vi "picoquant_write_processing_tasks.vi"(8 "error in (no error)":errorcluster, 10 "processing tasks":T1, 11 "picoquant_generic in":refnum<class "picoquant_generic.lvclass">) -> (0 "error out":errorcluster, 3 "picoquant_generic out":refnum<class "picoquant_generic.lvclass">)   [LabVIEW 2015, in "picoquant_generic.lvclass"]
uses:
  picoquant_generic.lvclass
  processing_tasks_tdef.ctl
  picoquant_generic.lvclass/picoquant_generic.ctl
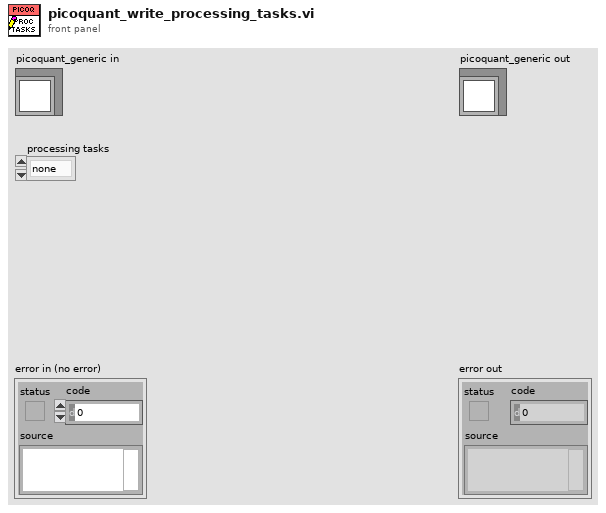
[diagram p1: front panel]
types:
  T1 = typedef "processing_tasks_tdef.ctl" = enum16{"none", "correlate", "histogram"}
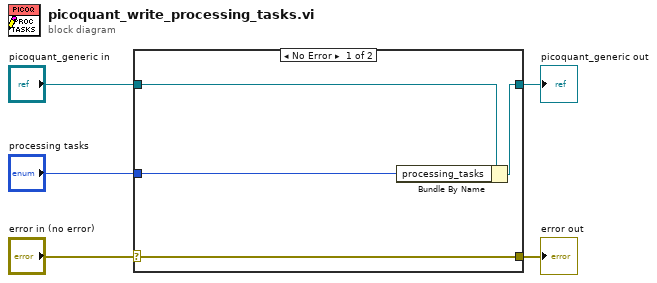
[diagram p0: block diagram]
diagram:
  n1 = case shown="No Error" "error in (no error)" {
    selector: "error in (no error)" -> [w9 w10]
    tunnel: [w9 w10] -> w4
    tunnel: [w7 w11] -> w2
    tunnel: "picoquant_generic in" -> [w8 w11]
    tunnel: "processing tasks" -> [w6 _]
    frame No Error {
      n2 = Bundle By Name(cluster=w8, "processing_tasks"=w6) -> (w7:refnum<class "picoquant_generic.lvclass">)
    }
    frame Error {
    }
  }
  "error out" <- w4
  "picoquant_generic out" <- w2
